vi "AutoDrive.vi"(9 "Steady Val":dbl, 11 "Distance to travel (inches)":dbl) -> ()   [LabVIEW 2012]
uses:
  StateMachineEnum.ctl
  Robot Global Data.vi
  <vilib>/Rock Robotics/WPI/RobotDrive/WPI_RobotDriveGetSetRefNum.vi
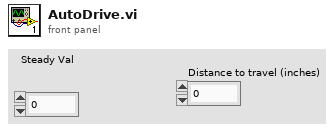
[diagram p1: front panel]
types:
  T1 = typedef "StateMachineEnum.ctl" = enum16{"Init", "Idle", "Start", "Do", "Stop"}
  T2 = typedef "WPI_EncoderDevRef.ctl" = cluster{"DevStatus":errorcluster, "EncoderIndex":T3, "CounterIndex":T4, "DistancePerCount":dbl, "Decoding Type":T5}
  T3 = typedef "FPGA_EncoderIdx.ctl" = enum8{"Enc 0", "Enc 1", "Enc 2", "Enc 3", "Invalid"}
  T4 = typedef "FPGA_CounterCtrSystemIndex.ctl" = enum8{"Ctr 0", "Ctr 1", "Ctr 2", "Ctr 3", "Ctr 4", "Ctr 5", "Ctr 6", "Ctr 7", "Invalid"}
  T5 = typedef "WPI_EncoderType.ctl" = enum16{"1x", "2x", "4x"}
  T6 = typedef "WPI_RobotDriveDevRef.ctl" = cluster{"DevStatus":errorcluster, "Motors[]":T7[], "Square Inputs":bool, "Max Output":dbl, "Isochronous":bool}
  T7 = typedef "WPI_MotorControlDeviceRef.ctl" = cluster{"DeviceStatus":errorcluster, "Type":enum16{"PWM", "CAN"}, "PWM":cluster{"Digital Module":T8, "PWM Channel":T9, "DeadBand":T10}, "CAN":cluster{"Device Number":u8, "Control Mode":T11, "Semaphore":T12, "Max Vout":dbl}, "Invert":bool, "TransformRef":T13, "InvTransformRef":T13}
  T8 = typedef "FPGA_TypedefDigitalModule.ctl" = enum16{"Digital Module 1", "Digital Module 2"}
  T9 = typedef "FPGA_DIOPWMChannel.ctl" = enum8{"PWM 1", "PWM 2", "PWM 3", "PWM 4", "PWM 5", "PWM 6", "PWM 7", "PWM 8", "PWM 9", "PWM 10", "Invalid"}
  T10 = typedef "WPI_PWMDeadband.ctl" = cluster{"Name":string, "maxPositivePwm":i32, "minPositivePwm":i32, "centerPwm":i32, "maxNegativePwm":i32, "minNegativePwm":i32, "angularRange":u16}
  T11 = typedef "WPI_CANJaguar_ControlMode.ctl" = enum8{"Percent VBus", "Current", "Speed", "Position", "Voltage"}
  T12 = typedef "Semaphore RefNum" = refnum<k1>
  T13 = typedef "WPI_PWMTransform_ConPane.ctl" = refnum<vi>
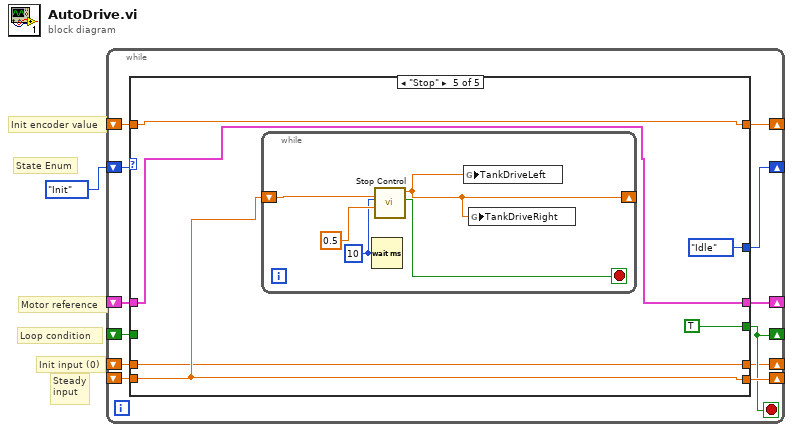
[diagram p0: block diagram]
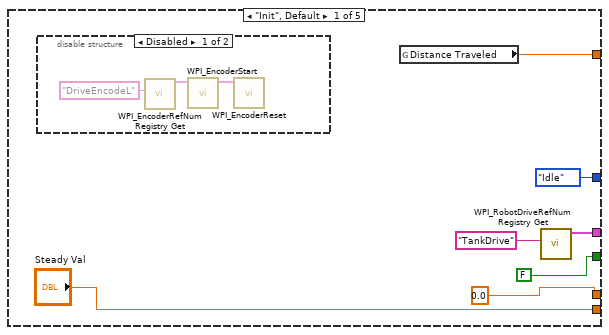
[diagram p2: hidden frame]
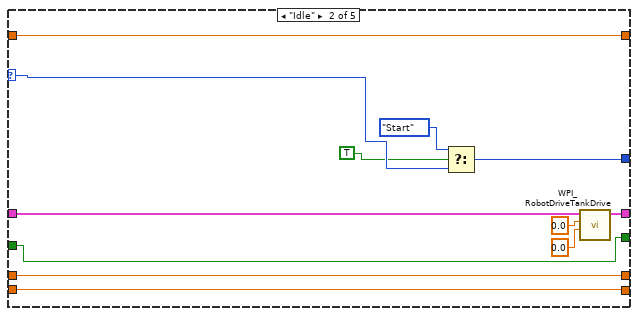
[diagram p4: hidden frame]
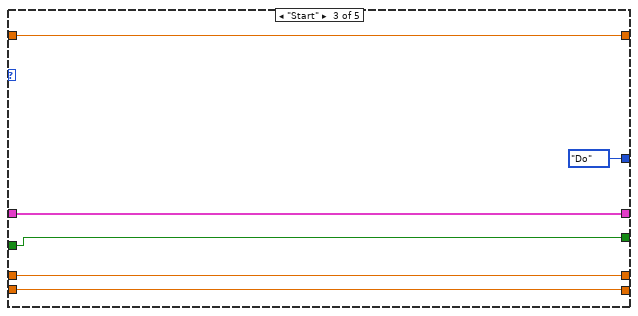
[diagram p5: hidden frame]
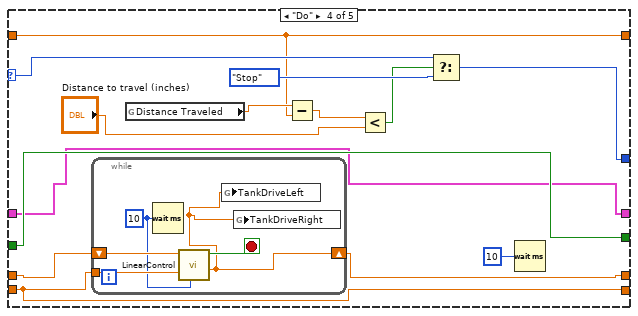
[diagram p6: hidden frame]
diagram:
  # "Init encoder value"
  # "State Enum"
  # "Motor reference"
  # "Loop condition"
  # "Init input (0)"
  # "Steady\ninput"
  n1 = while {
    shift-right: [w10] -> _
    shift-left: StateMachineEnum."Init" -> [w13]
    shift-right: [w12] -> _
    shift-left: _ -> [w11]
    shift-right: [w9] -> _
    shift-left: _ -> [w8]
    shift-right: [w7] -> _
    shift-left: _ -> [w6]
    shift-right: [w5] -> _
    shift-left: _ -> [w4]
    shift-right: [w3] -> _
    shift-left: _ -> [w2]
    stop <- w7 stop-if-true
    n2 = case shown="\"Stop\"" w13 {
      selector: w13 -> [_ w29 _ w55 _]
      tunnel: [w19 w30 w40 w45 w62] -> w12
      tunnel: w11 -> [_ w32 w40 w45 w62]
      tunnel: [StateMachineEnum."Idle" w35 StateMachineEnum."Do" w53 StateMachineEnum."Idle" ("f")] -> w10
      tunnel: ["Steady Val" w27 w39 w50 w65] -> w9
      tunnel: w8 -> [_ w27 w39 w50 w65]
      tunnel: [FALSE w26 w38 w48 TRUE] -> w7
      tunnel: w6 -> [_ w26 w38 w48 _]
      tunnel: [0.0 ("New Motor Input") w25 w37 w46 w63] -> w5
      tunnel: w4 -> [_ w25 w37 w47 w63]
      tunnel: [w14 w24 w36 w42 w61] -> w3
      tunnel: w2 -> [_ w24 w36 w42 w61]
      frame "Init", Default {
        n3 = disable-structure shown="Disabled" {
          frame Disabled {
            n4 = call <vilib>:"WPI_EncoderRefNum Registry Get.vi"("refnum name"="DriveEncodeL") -> ("EncoderDevRef"=w23:T2)  [unwired: 9 in, 1 out]
            n5 = call <vilib>:"WPI_EncoderStart.vi"("EncoderDevRef"=w23) -> ("EncoderDevRef"=w21:T2)  [unwired: 1 in, 9 out]
            n6 = call <vilib>:"WPI_EncoderReset.vi"("EncoderDevRef"=w21) -> ()  [unwired: 1 in, 10 out]
          }
          frame Enabled {
          }
        }
        n7 = global read "Robot Global Data.vi" "Distance Traveled"() -> (w14:dbl)
        n8 = call <vilib>:"WPI_RobotDriveRefNum Registry Get.vi"("refnum name"="TankDrive") -> ("RobotDriveDevRef"=w19:T6)  [unwired: 9 in, 1 out]
      }
      frame "Idle" {
        n9 = Select(t=StateMachineEnum."Start", s=TRUE, f=w29) -> (s? t:f=w35:T1)
        n10 = call <vilib>:"WPI_RobotDriveTankDrive.vi"("Right axis value"=0.0, "Left axis value"=0.0, "RobotDriveDevRef"=w32) -> ("RobotDriveDevRef"=w30:T6)  [unwired: 6 in, 2 out]
      }
      frame "Start" {
      }
      frame "Do" {
        n11 = while {
          shift-right: [w56] -> w46
          shift-left: w47 -> [w59]
          tunnel: w50 -> [w58]
          stop <- w60 stop-if-true
          w57 = u32 10 ("milliseconds to wait")
          n12 = Wait (ms)(milliseconds to wait=w57) -> ()  [unwired: 1 out]
          n13 = call "LinearControl.vi"("Loop Time (ms)"=w57, "Setpoint"=w58, "Recieved Motor Input"=w59) -> ("New Motor Input"=w56:dbl, "Currently Matching"=w60:bool)  [unwired: 7 in]
          n14 = global write "Robot Global Data.vi" "TankDriveLeft"(w56) -> ()
          n15 = global write "Robot Global Data.vi" "TankDriveRight"(w56) -> ()
        }
        n16 = global read "Robot Global Data.vi" "Distance Traveled"() -> (w44:dbl)
        n17 = Subtract(x=w44, y=w42) -> (x-y=w43:dbl)
        n18 = Less?(x=w43, y="Distance to travel (inches)") -> (x < y?=w51:bool)
        n19 = Select(t=w55, s=w51, f=StateMachineEnum."Stop") -> (s? t:f=w53:T1)
        n20 = Wait (ms)(milliseconds to wait=u32 10) -> ()  [unwired: 1 out]
      }
      frame "Stop" {
        n21 = while {
          shift-right: [w67] -> _
          shift-left: w65 -> [w70]
          stop <- w69 stop-if-true
          w68 = u32 10 ("milliseconds to wait")
          n22 = Wait (ms)(milliseconds to wait=w68) -> ()  [unwired: 1 out]
          n23 = call "Stop Control.vi"("Rate (unit/s)"=0.5, "Loop Time (ms)"=w68, "Recieved Motor Input"=w70) -> ("Done Stopping"=w69:bool, "New Motor Input"=w67:dbl)  [unwired: 7 in]
          n24 = global write "Robot Global Data.vi" "TankDriveLeft"(w67) -> ()
          n25 = global write "Robot Global Data.vi" "TankDriveRight"(w67) -> ()
        }
      }
    }
  }
